vi "CRC_16_MODBUS LUT_REFLECTED generator and test.vi"(1 "CRC init":u16=65535 format="%04x", 2 "Generating poly":u16=40961 min=1 format="%04x") -> (0 "CRC_16_MODBUS LUT_REFLECTED":u16[](array[numeric])=[0, 49345, 49537, 320, 49921, 960, 640, 49729, 50689, 1728, 1920, 51009, 1280, 50625, 50305, 1088, 52225, 3264, 3456, 52545, 3840, 53185, 52865, 3648, 2560, 51905, 52097, 2880, 51457, 2496, 2176, 51265, 55297, 6336, 6528, 55617, 6912, 56257, 55937, 6720, 7680, 57025, 57217, 8000, 56577, 7616, 7296, 56385, 5120, 54465, 54657, 5440, 55041, 6080, 5760, 54849, 53761, 4800, 4992, 54081, 4352, 53697, 53377, 4160, 61441, 12480, 12672, 61761, 13056, 62401, 62081, 12864, 13824, 63169, 63361, 14144, 62721, 13760, 13440, 62529, 15360, 64705, 64897, 15680, 65281, 16320, 16000, 65089, 64001, 15040, 15232, 64321, 14592, 63937, 63617, 14400, 10240, 59585, 59777, 10560, 60161, 11200, 10880, 59969, 60929, 11968, 12160, 61249, 11520, 60865, 60545, 11328, 58369, 9408, 9600, 58689, 9984, 59329, 59009, 9792, 8704, 58049, 58241, 9024, 57601, 8640, 8320, 57409, 40961, 24768, 24960, 41281, 25344, 41921, 41601, 25152, 26112, 42689, 42881, 26432, 42241, 26048, 25728, 42049, 27648, 44225, 44417, 27968, 44801, 28608, 28288, 44609, 43521, 27328, 27520, 43841, 26880, 43457, 43137, 26688, 30720, 47297, 47489, 31040, 47873, 31680, 31360, 47681, 48641, 32448, 32640, 48961, 32000, 48577, 48257, 31808, 46081, 29888, 30080, 46401, 30464, 47041, 46721, 30272, 29184, 45761, 45953, 29504, 45313, 29120, 28800, 45121, 20480, 37057, 37249, 20800, 37633, 21440, 21120, 37441, 38401, 22208, 22400, 38721, 21760, 38337, 38017, 21568, 39937, 23744, 23936, 40257, 24320, 40897, 40577, 24128, 23040, 39617, 39809, 23360, 39169, 22976, 22656, 38977, 34817, 18624, 18816, 35137, 19200, 35777, 35457, 19008, 19968, 36545, 36737, 20288, 36097, 19904, 19584, 35905, 17408, 33985, 34177, 17728, 34561, 18368, 18048, 34369, 33281, 17088, 17280, 33601, 16640, 33217, 32897, 16448] format="%04x")   [LabVIEW 2020]
doc: "Modbus RTU for Invertek drives. Paul Nathan 21-JUN-2022."
panel:
  out "Pass":bool=TRUE
  out "CRC":u16=39985 format="%04x"
  in  "Answer":u16=39985 format="%04x"
  in  "Test":u16=48879 format="%04x"
  out "CRC_16 LUT":string="0x0000, 0xC0C1, 0xC181, 0x0140, 0xC301, 0x03C0, 0x0280, 0xC241, 0xC601, 0x06C0, 0x0780, 0xC741, 0x0500, 0xC5C1, 0xC481, 0x0440, \r\n0xCC01, 0x0CC0, 0x0D80, 0xCD41, 0x0F00, 0xCFC1, 0xCE81, 0x0E40, 0x0A00, 0xCAC1, 0xCB81, 0x0B40, 0xC901, 0x09C0, 0x0880, 0xC841, \r\n0xD801, 0x18C0, 0x1980, 0xD941, 0x1B00, 0xDBC1, 0xDA81, 0x1A40, 0x1E00, 0xDEC1, 0xDF81, 0x1F40, 0xDD01, 0x1DC0, 0x1C80, 0xDC41, \r\n0x1400, 0xD4C1, 0xD581, 0x1540, 0xD701, 0x17C0, 0x1680, 0xD641, 0xD201, 0x12C0, 0x1380, 0xD341, 0x1100, 0xD1C1, 0xD081, 0x1040, \r\n0xF001, 0x30C0, 0x3180, 0xF141, 0x3300, 0xF3C1, 0xF281, 0x3240, 0x3600, 0xF6C1, 0xF781, 0x3740, 0xF501, 0x35C0, 0x3480, 0xF441, \r\n0x3C00, 0xFCC1, 0xFD81, 0x3D40, 0xFF01, 0x3FC0, 0x3E80, 0xFE41, 0xFA01, 0x3AC0, 0x3B80, 0xFB41, 0x3900, 0xF9C1, 0xF881, 0x3840, \r\n0x2800, 0xE8C1, 0xE981, 0x2940, 0xEB01, 0x2BC0, 0x2A80, 0xEA41, 0xEE01, 0x2EC0, 0x2F80, 0xEF41, 0x2D00, 0xEDC1, 0xEC81, 0x2C40, \r\n0xE401, 0x24C0, 0x2580, 0xE541, 0x2700, 0xE7C1, 0xE681, 0x2640, 0x2200, 0xE2C1, 0xE381, 0x2340, 0xE101, 0x21C0, 0x2080, 0xE041, \r\n0xA001, 0x60C0, 0x6180, 0xA141, 0x6300, 0xA3C1, 0xA281, 0x6240, 0x6600, 0xA6C1, 0xA781, 0x6740, 0xA501, 0x65C0, 0x6480, 0xA441, \r\n0x6C00, 0xACC1, 0xAD81, 0x6D40, 0xAF01, 0x6FC0, 0x6E80, 0xAE41, 0xAA01, 0x6AC0, 0x6B80, 0xAB41, 0x6900, 0xA9C1, 0xA881, 0x6840, \r\n0x7800, 0xB8C1, 0xB981, 0x7940, 0xBB01, 0x7BC0, 0x7A80, 0xBA41, 0xBE01, 0x7EC0, 0x7F80, 0xBF41, 0x7D00, 0xBDC1, 0xBC81, 0x7C40, \r\n0xB401, 0x74C0, 0x7580, 0xB541, 0x7700, 0xB7C1, 0xB681, 0x7640, 0x7200, 0xB2C1, 0xB381, 0x7340, 0xB101, 0x71C0, 0x7080, 0xB041, \r\n0x5000, 0x90C1, 0x9181, 0x5140, 0x9301, 0x53C0, 0x5280, 0x9241, 0x9601, 0x56C0, 0x5780, 0x9741, 0x5500, 0x95C1, 0x9481, 0x5440, \r\n0x9C01, 0x5CC0, 0x5D80, 0x9D41, 0x5F00, 0x9FC1, 0x9E81, 0x5E40, 0x5A00, 0x9AC1, 0x9B81, 0x5B40, 0x9901, 0x59C0, 0x5880, 0x9841, \r\n0x8801, 0x48C0, 0x4980, 0x8941, 0x4B00, 0x8BC1, 0x8A81, 0x4A40, 0x4E00, 0x8EC1, 0x8F81, 0x4F40, 0x8D01, 0x4DC0, 0x4C80, 0x8C41, \r\n0x4400, 0x84C1, 0x8581, 0x4540, 0x8701, 0x47C0, 0x4680, 0x8641, 0x8201, 0x42C0, 0x4380, 0x8341, 0x4100, 0x81C1, 0x8081, 0x4040"
  # "This VI is for reference only and shows how the Modbus CRC LUT is generated and how the CRC is computed."
  # "Drag this 1D array into a block diagram to use as a MODBUS CRC LUT const."
  # "PN 21-06-2022"
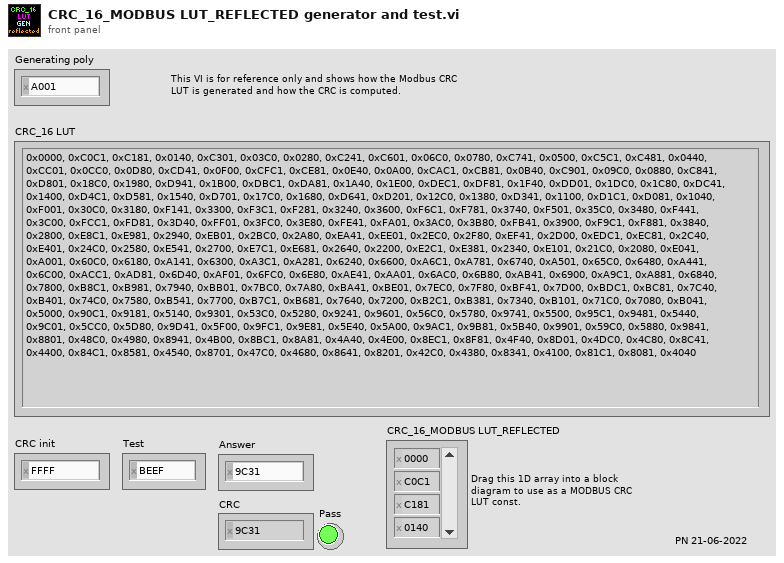
[diagram p1: front panel]
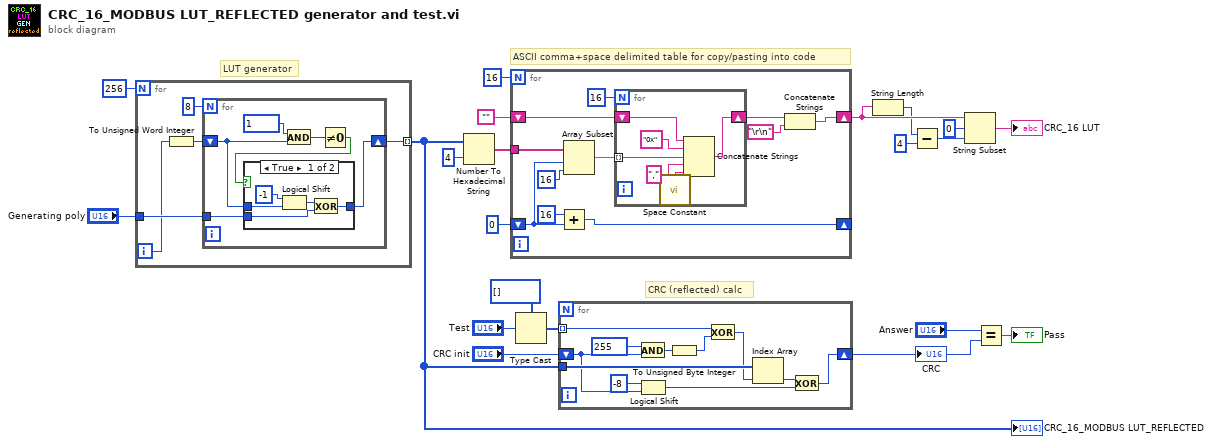
[diagram p0: block diagram]
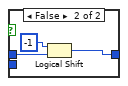
[diagram p2: hidden frame]
diagram:
  # "CRC (reflected) calc"
  # "ASCII comma+space delimited table for copy/pasting into code"
  # "LUT generator"
  n1 = for {
    N: 256 -> [_]
    tunnel: "Generating poly" -> [w25]
    tunnel: [w24] -> w1 mode=indexing
    i -> [w22]
    n2 = To Unsigned Word Integer(number=w22) -> (unsigned 16bit integer=w23:u16)
    n3 = for {
      N: 8 -> [_]
      tunnel: w25 -> [w28]
      shift-right: [w27] -> w24
      shift-left: w23 -> [w29]
      n4 = And(x=u16 1 ("y"), y=w29) -> (x .and. y?=w31:u16)
      n5 = Not Equal To 0?(x=w31) -> (x != 0?=w30:bool)
      n6 = case shown="True" w30 {
        tunnel: w29 -> [w36 w39]
        tunnel: w28 -> [w35 _]
        tunnel: [w34 w38] -> w27
        frame True {
          n7 = Logical Shift(y=i16 -1, x=w36) -> (x << y=w33:u16)
          n8 = Exclusive Or(1:w35, 2:w33) -> (0:w34:u16)
        }
        frame False {
          n9 = Logical Shift(y=i16 -1, x=w39) -> (x << y=w38:u16)
        }
      }
    }
  }
  "CRC_16_MODBUS LUT_REFLECTED" <- w1
  n10 = Number To Hexadecimal String(1:i16 4 ("width (-)"), 2:w1) -> (0:w20:string[])
  n11 = for {
    N: 16 -> [_]
    tunnel: w20 -> [w49]
    shift-right: [w50] -> _
    shift-left: 0 -> [w48]
    shift-right: [w42] -> w16
    shift-left: "" -> [w41]
    n12 = Add(x=16, y=w48) -> (x+y=w50:i32)
    n13 = Array Subset(array=w49, index=w48, length=16) -> (w46:string[])
    n14 = for {
      N: 16 -> [_]
      tunnel: w46 -> [w56] mode=indexing
      shift-right: [w54] -> w44
      shift-left: w41 -> [w55]
      n15 = call <vilib>:"Space Constant.vi"() -> ("String"=w52:string)
      n16 = Concatenate Strings(w55, "0x" ("string"), w56, "," ("string"), w52) -> (w54:string)
    }
    n17 = Concatenate Strings(w44, "\r\n") -> (w42:string)
  }
  n18 = Type Cast(type=u8[] [], x="Test") -> (*(type *) &x=w2:u8[])
  n19 = for {
    tunnel: w2 -> [w61] mode=indexing
    tunnel: w1 -> [w68]
    shift-right: [w64] -> w3
    shift-left: "CRC init" -> [w62]
    n20 = And(x=u16 255 ("y"), y=w62) -> (x .and. y?=w60:u16)
    n21 = Logical Shift(y=i16 -8, x=w62) -> (x << y=w65:u16)
    n22 = To Unsigned Byte Integer(number=w60) -> (unsigned 8bit integer=w59:u8)
    n23 = Exclusive Or(1:w59, 2:w61) -> (0:w58:u8)
    n24 = Index Array(array=w68, index=w58) -> (element=w67:u16)
    n25 = Exclusive Or(1:w65, 2:w67) -> (0:w64:u16)
  }
  "CRC" <- w3
  n26 = String Length(string=w16) -> (length=w13:i32)
  n27 = Subtract(x=w13, y=4) -> (x-y=w12:i32)
  n28 = String Subset(string=w16, offset (0)=0, length (rest)=w12) -> (substring=→"CRC_16 LUT":string)
  n29 = Equal?(x="Answer", y=w3) -> (x = y?=→"Pass":bool)
